vi "getPathOfTestMonitor.vi"() -> (3 "testMonitorPath":path)   [LabVIEW 2018]
doc: "Get the path of test monitor of SAL."
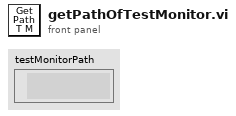
[diagram p1: front panel]
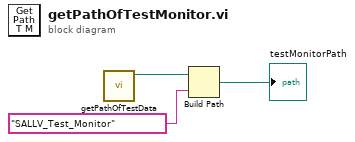
[diagram p0: block diagram]
diagram:
  n1 = call "getPathOfTestData.vi"() -> ("testDataPath"=w3:path)  [unwired: 11 in]
  n2 = Build Path(base path=w3, name or relative path="SALLV_Test_Monitor") -> (appended path=→"testMonitorPath":path)
